vi "SYST_SHOR_EXEC.vi"(0 "VISA IN":refnum<visa-resource-name>, 5 "error in":errorcluster, 7 "Number":i32) -> (14 "VISA Out":refnum<visa-resource-name>, 19 "error out":errorcluster)   [LabVIEW 2018, in "PNA-X.lvlib"]
doc: "SYSTem:SHORtcut<n>:EXECute \n1882\n\n(Write-only) Executes (runs) the specified Macro (shortcut) that is stored in the PNA. \nParameters \n<n> Numeric. Number of the macro that is stored in the PNA. \nTo find the number of a macro, either open the Macro Setup dialog and count \nthe line number of the desired macro, or query the titles of all 12 macros for the \ndesired macro title. \nExamples SYST:SHOR1:EXEC \nQuery Syntax Not Applicable \nDefault Not Applicable"
uses:
  PNA-X.lvlib
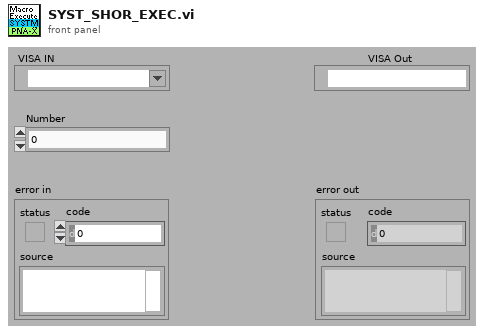
[diagram p1: front panel]
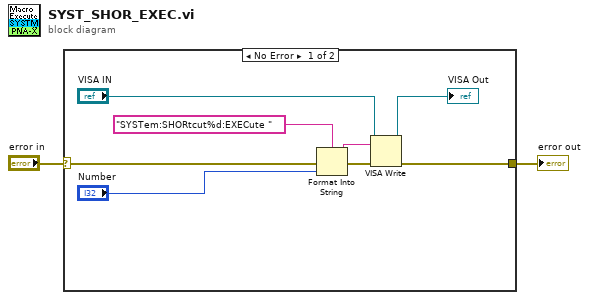
[diagram p0: block diagram]
diagram:
  n1 = case shown="No Error" "error in" {
    selector: "error in" -> [w10 w11]
    tunnel: [w5 w11] -> w1
    frame No Error {
      n2 = Format Into String(format string="SYSTem:SHORtcut%d:EXECute " ("Cmdline"), error in=w10, "Number") -> (resulting string=w8:string, error out=w9:errorcluster)  [unwired: 1 in]
      n3 = VISA Write(VISA resource name="VISA IN", write buffer=w8, error in (no error)=w9) -> (VISA resource name out=→"VISA Out":refnum<visa-resource-name>, error out=w5:errorcluster)  [unwired: 1 out]
    }
    frame Error {
    }
  }
  "error out" <- w1
